vi "FisherPaykel Wash State Setup.vi"(7 "Agitate Parameters Settle Stroke":T1={"Agitate Running Time (sec)"=15, "Direction (CW or CCW)"="1", "RampUpTime (1-600ms)"=250, "TargetSpeed (0-200RPM)"=726, "PlateauTime (0-1800ms 10ms Increment)"=1000, "PauseTime (0-1800ms 10ms Increment)"=600} {"PauseTime (0-1800ms 10ms Increment)" step=10; "PlateauTime (0-1800ms 10ms Increment)" step=10; "TargetSpeed (0-200RPM)" max=1600 step=1; "RampUpTime (1-600ms)" max=600 step=10; "Agitate Running Time (sec)" step=1}, 8 "error in (no error)":errorcluster, 9 "Motor Profile Data":T4, 10 "Spin Profile in":T3 {"Running Time (s)" step=1; "Acceleration Rate - (10 Slowest/1000 Fastest)" min=10 max=1000 step=1; "Target Speed (RPM)" min=23 max=1600 step=1}, 11 "Agitate Parameters in":T1 {"PauseTime (0-1800ms 10ms Increment)" step=10; "PlateauTime (0-1800ms 10ms Increment)" step=10; "TargetSpeed (0-200RPM)" max=1600 step=1; "RampUpTime (1-600ms)" max=600 step=10; "Agitate Running Time (sec)" step=1}) -> (0 "error out":errorcluster, 2 "Spin Profile out":T3 {"Running Time (s)" step=1; "Acceleration Rate - (10 Slowest/1000 Fastest)" min=10 max=1000 step=1; "Target Speed (RPM)" min=23 max=1600 step=1}, 3 "Agitate Parameters out":T1 {"PauseTime (0-1800ms 10ms Increment)" step=10; "PlateauTime (0-1800ms 10ms Increment)" step=10; "TargetSpeed (0-200RPM)" max=1600 step=1; "RampUpTime (1-600ms)" max=600 step=10; "Agitate Running Time (sec)" step=1}, 5 "States Out":string)   [LabVIEW 2016]
uses:
  Type Definitions/FisherPaykel Motor Profile Data ERD.ctl
  Type Definitions/Fisher Paykel Motor Profile.ctl
  Type Definitions/FisherPaykel Direction CMD.ctl
  Type Definitions/Fisher Paykel Agitate Parameters.ctl
panel:
  # "Agitate Profile Parameters"
  # "Agitate Start Parameters"
  # "Agitate Profile Parameters"
  # "Agitate Start Parameters"
  # "Agitate Profile Parameters"
  # "Agitate Start Parameters"
  # "Spin Profile Parameters"
  # "Spin Start Parameters"
  # "Spin Profile Parameters"
  # "Spin Start Parameters"
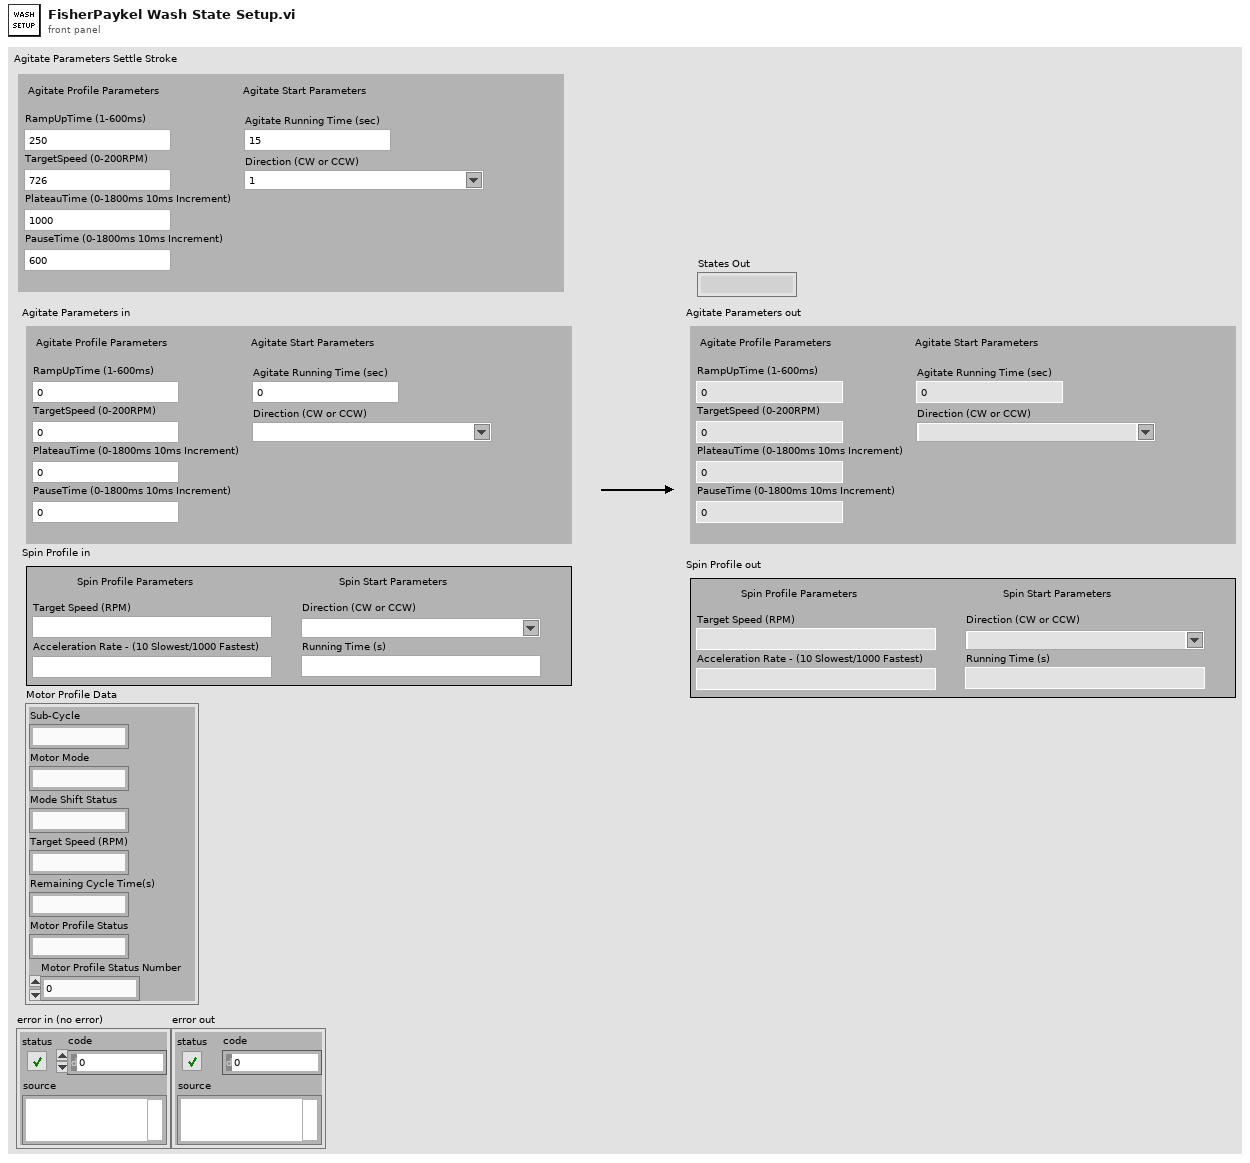
[diagram p1: front panel]
types:
  T1 = typedef "Fisher Paykel Agitate Parameters.ctl" = cluster{"Agitate Running Time (sec)":u16, "Direction (CW or CCW)":T2, "RampUpTime (1-600ms)":u16, "TargetSpeed (0-200RPM)":u16, "PlateauTime (0-1800ms 10ms Increment)":u16, "PauseTime (0-1800ms 10ms Increment)":u16}
  T2 = typedef "FisherPaykel Direction CMD.ctl" = string
  T3 = typedef "Fisher Paykel Motor Profile.ctl" = cluster{"Target Speed (RPM)":u16, "Acceleration Rate - (10 Slowest/1000 Fastest)":u16, "Running Time (s)":u16, "Direction (CW or CCW)":T2}
  T4 = typedef "FisherPaykel Motor Profile Data ERD.ctl" = cluster{"Sub-Cycle":string, "Motor Mode":string, "Mode Shift Status":string, "Target Speed (RPM)":string, "Remaining Cycle Time(s)":string, "Motor Profile Status":string, "Motor Profile Status Number":u16}
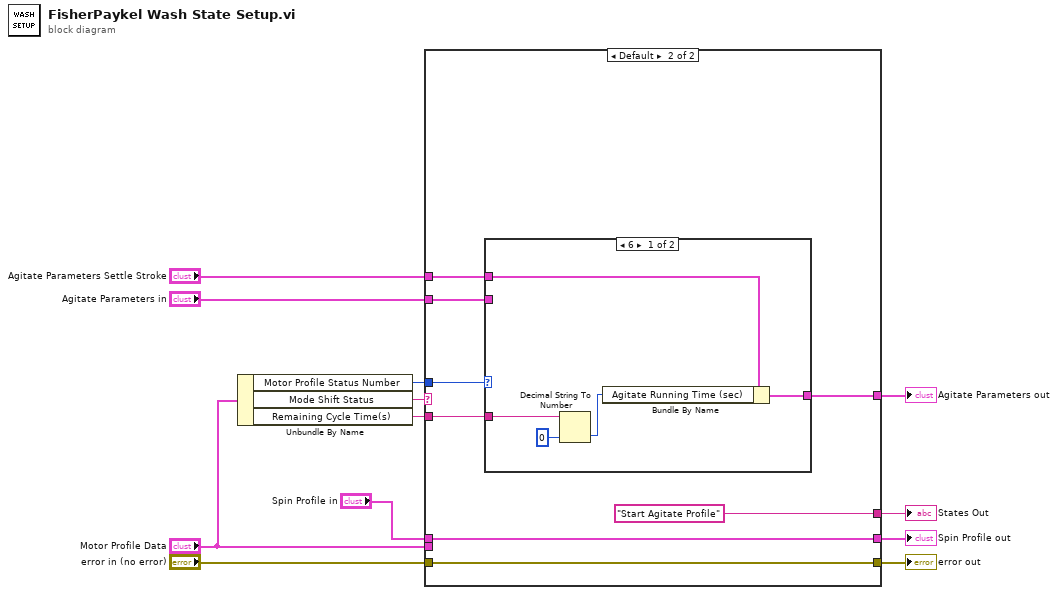
[diagram p0: block diagram]
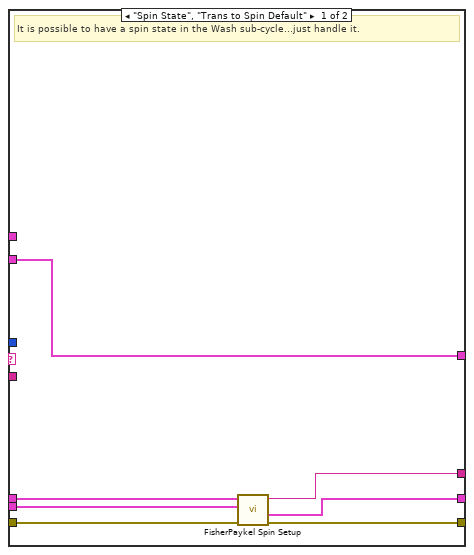
[diagram p2: hidden frame]
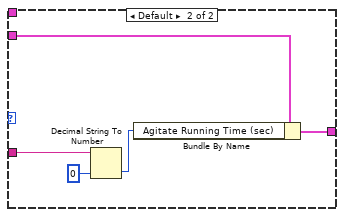
[diagram p3: hidden frame]
diagram:
  n1 = Unbundle By Name("Motor Profile Data") -> ("Motor Profile Status Number"=w2:u16, "Mode Shift Status"=w4:string, "Remaining Cycle Time(s)"=w3:string)
  n2 = case shown="Default" w4 {
    tunnel: [w17 "Start Agitate Profile"] -> w6
    tunnel: "Agitate Parameters in" -> [w16 w26]
    tunnel: [w16 w25] -> w8
    tunnel: "Spin Profile in" -> [w19 w24]
    tunnel: [w18 w24] -> w10
    tunnel: "error in (no error)" -> [w15 w23]
    tunnel: [w14 w23] -> w12
    tunnel: "Motor Profile Data" -> [w13 _]
    tunnel: w3 -> [_ w22]
    tunnel: w2 -> [_ w21]
    tunnel: "Agitate Parameters Settle Stroke" -> [_ w20]
    frame "Spin State", "Trans to Spin Default" {
      # "It is possible to have a spin state in the Wash sub-cycle...just handle it."
      n3 = call "FisherPaykel Spin Setup.vi"("Error In"=w15, "Motor Profile Data"=w13, "Spin Profile in"=w19) -> ("Error Out"=w14:errorcluster, "Spin Profile out"=w18:T3, "States Out"=w17:string)  [unwired: 6 in]
    }
    frame Default {
      n4 = case shown="6" w21 {
        tunnel: w26 -> [_ w37]
        tunnel: [w28 w36] -> w25
        tunnel: w22 -> [w30 w33]
        tunnel: w20 -> [w29 _]
        frame 6 {
          n5 = Decimal String To Number(string=w30, default (0L)=u16 0 ("default (0 I32)")) -> (number=w31:u16)  [unwired: 1 in, 1 out]
          n6 = Bundle By Name(cluster=w29, "Agitate Running Time (sec)"=w31) -> (w28:T1)
        }
        frame Default {
          n7 = Decimal String To Number(string=w33, default (0L)=u16 0 ("default (0 I32)")) -> (number=w34:u16)  [unwired: 1 in, 1 out]
          n8 = Bundle By Name(cluster=w37, "Agitate Running Time (sec)"=w34) -> (w36:T1)
        }
      }
    }
  }
  "error out" <- w12
  "Spin Profile out" <- w10
  "Agitate Parameters out" <- w8
  "States Out" <- w6
